vi "Save Image.vi"(8 "error in (no error)":errorcluster, 10 "path":string, 11 "CCDCamera in":refnum<class "CCDCamera.lvclass">) -> (0 "error out":errorcluster, 3 "CCDCamera out":refnum<class "CCDCamera.lvclass">)   [LabVIEW 2018, in "CCDCamera.lvclass"]
uses:
  CCDCamera.lvclass
  <userlib>/atmcd32d.llb/FITS_type typedef.ctl
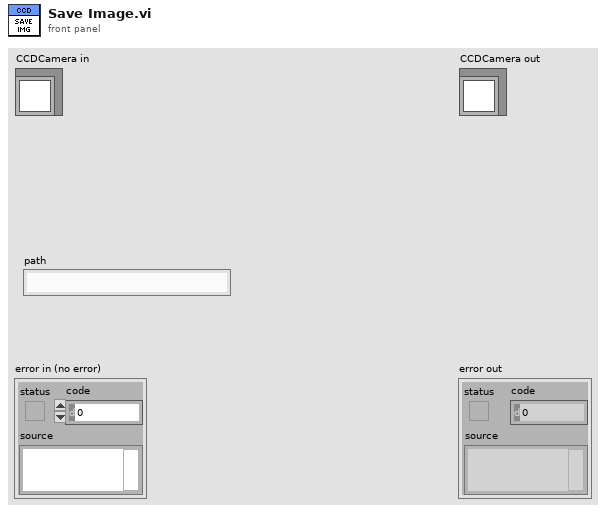
[diagram p1: front panel]
types:
  T1 = typedef "FITS_type typedef.ctl" = enum16{"Unsigned 16", "Unsigned 32", "Signed 16", "Signed 32", "Float"}
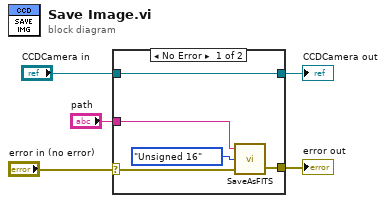
[diagram p0: block diagram]
diagram:
  n1 = case shown="No Error" "error in (no error)" {
    selector: "error in (no error)" -> [w9 w12]
    tunnel: [w8 w12] -> w4
    tunnel: [w10 w11] -> w2
    tunnel: "CCDCamera in" -> [w10 w11]
    tunnel: "path" -> [w6 _]
    frame No Error {
      n2 = call <userlib>:"SaveAsFITS.vi"("error in (no error)"=w9, "FITS_type"=FITS_type_typedef."Unsigned 16", "path"=w6) -> ("error out"=w8:errorcluster)  [unwired: 1 out]
    }
    frame Error {
    }
  }
  "error out" <- w4
  "CCDCamera out" <- w2
